vi "Open.vi"(8 "error in (no error)":errorcluster, 11 "subprocess in":refnum<class "Subprocess.lvclass">) -> (0 "error out":errorcluster, 3 "subprocess out":refnum<class "Subprocess.lvclass">)   [LabVIEW 2020, in "NI_Subprocess.lvlib" / "Subprocess.lvclass"]
doc: "Execute the configured command. Use <b>subprocess out</b> to interact with the running command."
uses:
  <vilib>/Subprocess/Subprocess/Subprocess.lvclass
  <vilib>/Subprocess/Subprocess/Subprocess.lvclass/Subprocess.ctl
  lviosrg.dll
  <vilib>/Utility/error.llb/Error Cluster From Error Code.vi
  <vilib>/ErrorRing/Error Ring.xnode
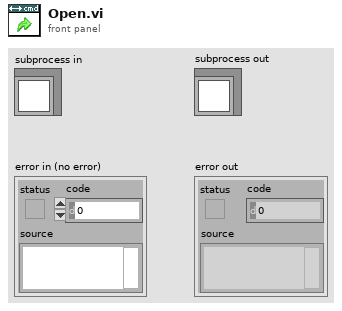
[diagram p1: front panel]
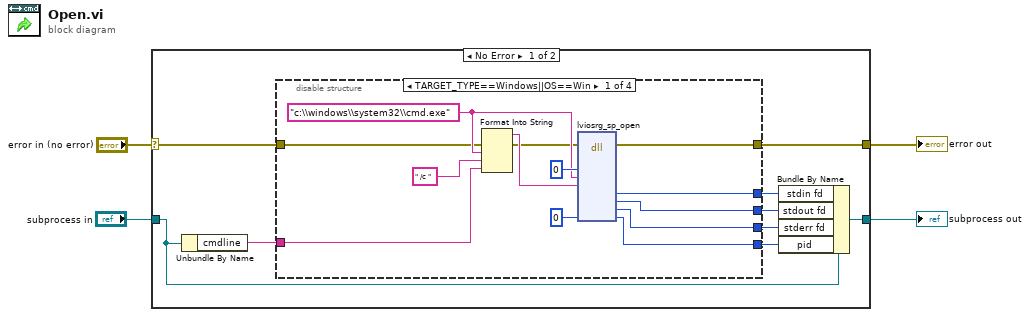
[diagram p0: block diagram]
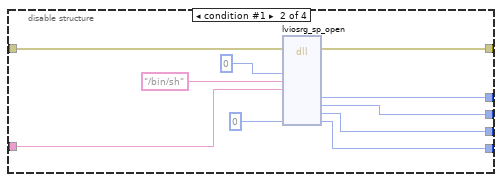
[diagram p2: hidden frame]
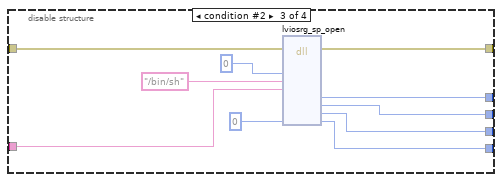
[diagram p3: hidden frame]
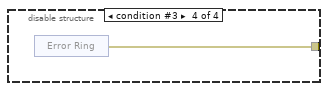
[diagram p4: hidden frame]
diagram:
  n1 = case shown="No Error" "error in (no error)" {
    selector: "error in (no error)" -> [w13 w53]
    tunnel: [w12 w53] -> w3
    tunnel: [w6 w52] -> w2
    tunnel: "subprocess in" -> [w11 w52]
    frame No Error {
      n2 = Unbundle By Name(w11) -> ("cmdline"=w5:string)
      n3 = disable-structure shown="TARGET_TYPE==Windows||OS==Win" {
        disable-tunnel: w13 -> [w19 w35 w45 _]
        disable-tunnel: [w25 w34 w44 w47] -> w12
        disable-tunnel: [w18 w31 w41 _] -> w10
        disable-tunnel: [w17 w30 w40 _] -> w9
        disable-tunnel: [w16 w29 w39 _] -> w8
        disable-tunnel: [w15 w28 w38 _] -> w7
        disable-tunnel: w5 -> [w14 w27 w37 _]
        frame condition #0 (active) {
          w22 = "c:\\windows\\system32\\cmd.exe"
          n4 = Format Into String(error in=w19, w22, " /c " ("input 2"), w14) -> (resulting string=w23:string, error out=w20:errorcluster)  [unwired: 2 in]
          n5 = dll-call lib="lviosrg.*" fn="lviosrg_sp_open"(error in=w20, "errno"=0, "cmd"=w22, "args"=w23, "pb"=u64 0) -> (error out=w25:errorcluster, "fd_stdin"=w18:u64, "fd_stdout"=w17:u64, "fd_stderr"=w16:u64, "pb"=w15:u64)  [unwired: 11 in, 1 out]
        }
        frame condition #1 {
          n6 = dll-call lib="lviosrg.*" fn="lviosrg_sp_open"(error in=w35, "errno"=0, "cmd"="/bin/sh", "args"=w27, "pb"=u64 0) -> (error out=w34:errorcluster, "fd_stdin"=w31:u64, "fd_stdout"=w30:u64, "fd_stderr"=w29:u64, "pb"=w28:u64)  [unwired: 11 in, 1 out]
        }
        frame condition #2 {
          n7 = dll-call lib="lviosrg.*" fn="lviosrg_sp_open"(error in=w45, "errno"=0, "cmd"="/bin/sh", "args"=w37, "pb"=u64 0) -> (error out=w44:errorcluster, "fd_stdin"=w41:u64, "fd_stdout"=w40:u64, "fd_stderr"=w39:u64, "pb"=w38:u64)  [unwired: 11 in, 1 out]
        }
        frame condition #3 {
          n8 = xnode "Error Ring"() -> ("error out"=w47:errorcluster)
        }
      }
      n9 = Bundle By Name(cluster=w11, "stdin fd"=w10, "stdout fd"=w9, "stderr fd"=w8, "pid"=w7) -> (w6:refnum<class "Subprocess.lvclass">)
    }
    frame Error {
    }
  }
  "error out" <- w3
  "subprocess out" <- w2
